vi "Construct - File.vi"(6 "Console Ref":refnum<vi>, 10 "section":string, 11 "config file":path) -> (0 "Error Out":errorcluster, 3 "Sink-Console":refnum<class "Sink-Console.lvclass">)   [LabVIEW 2019, in "TSC Event Logger.lvlib" / "Sink-Console.lvclass"]
doc: "Create the sink for a console from ini file loading.\n\n<b>Code Developed By:</b>\nTechnology Service Corporation\nBloomington, IN 47403\nwww.tsc.com/atcs\n\nDeveloper:\nDaniel Coons"
uses:
  Sink-Console.lvclass
  C:/Development/Open Source/tsc-event-logger/Log Sinks/Log Sinks.lvclass
  Sink-Console.lvclass/Sink-Console.ctl
  <vilib>/Utility/config.llb/Read Key (I32).vi
  <vilib>/Utility/config.llb/NI_LVConfig.lvlib
  Log Sinks.lvclass
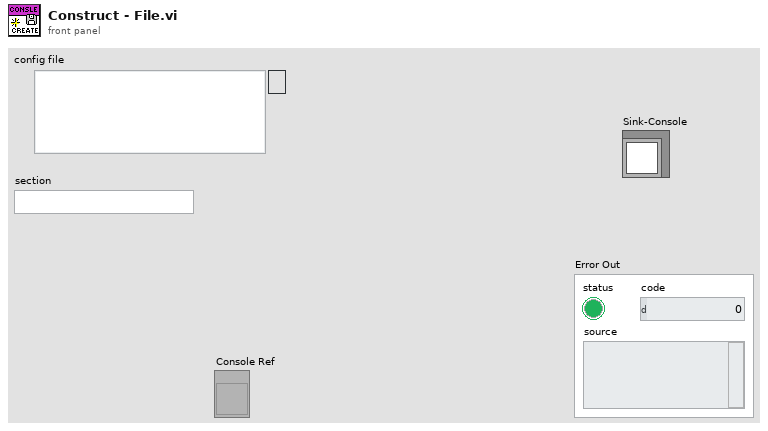
[diagram p1: front panel]
types:
  T1 = typedef "NI_LVConfig.lvlib/Config Data RefNum.ctl" = refnum<k1>
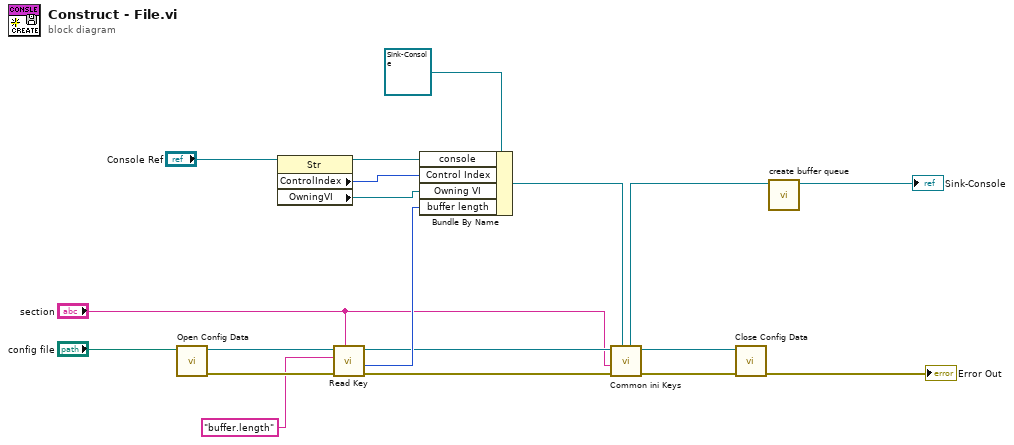
[diagram p0: block diagram]
diagram:
  n1 = call <vilib>:"Open Config Data.vi"("configuration file path"="config file") -> ("error out"=w14:errorcluster, "refnum"=w11:T1)  [unwired: 8 in, 1 out]
  n2 = property class="Str"(reference="Console Ref") -> (reference out=w15:refnum<vi>, "ControlIndex"=w16:i32, "OwningVI"=w17:refnum<vi>)  [unwired: 1 in, 1 out]
  n3 = call-poly <vilib>:"Read Key.vi"("section"="section", "error in (no error)"=w14, "key"="buffer.length", "refnum"=w11) -> ("error out"=w7:errorcluster, "value"=w9:i32, "refnum out"=w5:T1)  [unwired: 4 in, 1 out]
  n4 = Bundle By Name(cluster=refnum<class "Sink-Console.lvclass"> refnum ("TSC Event Logger.lvlib:Sink-Console.lvclass"), "console"=w15, "Control Index"=w16, "Owning VI"=w17, "buffer length"=w9) -> (w3:refnum<class "Sink-Console.lvclass">)
  n5 = call "Common ini Keys.vi"("Log Sinks in"=w3, "error in (no error)"=w7, "section"="section", "refnum in"=w5) -> ("error out"=w6:errorcluster, "refnum out"=w4:T1, "Log Sinks out"=w2:refnum<class "Sink-Console.lvclass">)  [unwired: 5 in]
  n6 = call <vilib>:"Close Config Data.vi"("error in (no error)"=w6, "refnum"=w4) -> ("error out"=→"Error Out":errorcluster)  [unwired: 8 in, 1 out]
  n7 = call "create buffer queue.vi"("Sink-Console in"=w2) -> ("Sink-Console out"=→"Sink-Console":refnum<class "Sink-Console.lvclass">)  [unwired: 9 in, 1 out]
